vi "setVoltage.vi"(7 "chn":string, 8 "error in (no error)":errorcluster, 10 "Voltage":dbl, 11 "PsTti in":refnum<class "PsuTti.lvclass">) -> (0 "error out":errorcluster, 3 "PsTti out":refnum<class "PsuTti.lvclass">)   [LabVIEW 2023, in "PsuTti.lvclass"]
doc: "set output voltage of the powersupply channel"
uses:
  PsuTti.lvclass
  PsuTti.lvclass/PsuTti.ctl
  driver/Tti-Pl303Qmd.lvlib
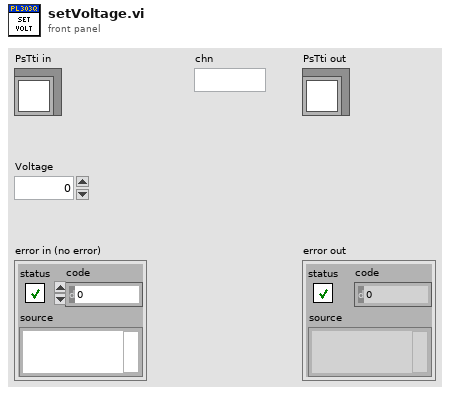
[diagram p1: front panel]
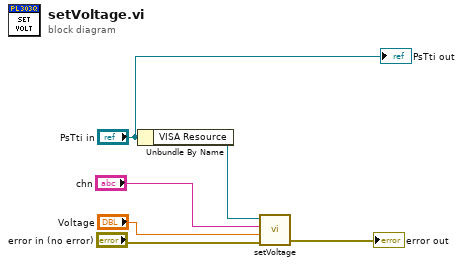
[diagram p0: block diagram]
diagram:
  n1 = Unbundle By Name("PsTti in") -> ("VISA Resource"=w2:refnum<visa-resource-name>)
  n2 = call "setVoltage.vi"("error in (no error)"="error in (no error)", "Voltage in Volts (1)"="Voltage", "Channel Nr (1)"="chn", "VISA resource name"=w2) -> ("error out"=→"error out":errorcluster)  [unwired: 6 in, 1 out]
  "PsTti out" <- "PsTti in"
